vi "UTIL_Round_100.vi"(7 "Num Refnum":refnum<vi>, 10 "100":bool, 11 "IN":dbl) -> (3 "OUT":dbl)   [LabVIEW 2024]
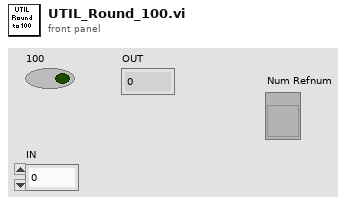
[diagram p1: front panel]
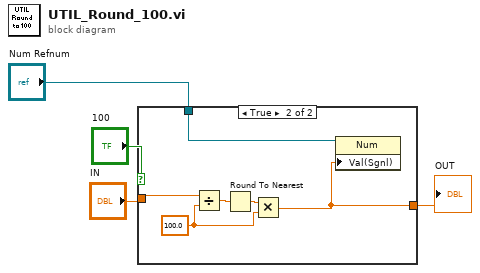
[diagram p0: block diagram]
diagram:
  n1 = case shown="True" "100" {
    tunnel: [w5 w6] -> w3
    tunnel: "IN" -> [w5 w8]
    tunnel: "Num Refnum" -> [_ w7]
    frame False {
    }
    frame True {
      w9 = 100.0 ("y")
      n2 = Divide(x=w8, y=w9) -> (x/y=w10:dbl)
      n3 = Round To Nearest(number=w10) -> (nearest integer value=w11:dbl)
      n4 = Multiply(x=w11, y=w9) -> (x*y=w6:dbl)
      n5 = property class="Num"(reference=w7, "Val(Sgnl)"=w6) -> ()  [unwired: 1 in, 2 out]
    }
  }
  "OUT" <- w3
